vi "sedSpectrometer_acceptCommand_setSpectTempSetpoint.vi"(8 "error in (no error)":errorcluster, 11 "command_setSpectTempSetpoint_Ctl":T1) -> (0 "error out":errorcluster, 2 "function return":i32, 3 "command_setSpectTempSetpoint_Ctl out":T1)   [LabVIEW 2016, in "SALLV_sedSpectrometer.lvlib"]
doc: "int sedSpectrometer_shm_acceptCommand_setSpectTempSetpointLV(sedSpectrometer_command_setSpectTempSetpointLV *command_setSpectTempSetpoint_Ctl );"
uses:
  SALLV_sedSpectrometer.lvlib
  DataTypes/command_setSpectTempSetpoint.ctl
  SALLV_sedSpectrometer.so
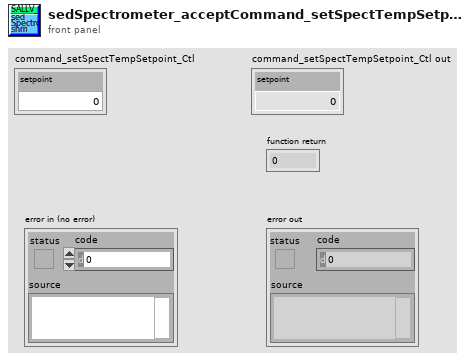
[diagram p1: front panel]
types:
  T1 = typedef "SALLV_sedSpectrometer.lvlib/command_setSpectTempSetpoint.ctl" = cluster{"setpoint":sgl}
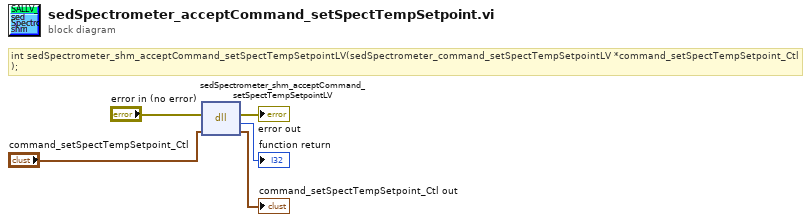
[diagram p0: block diagram]
diagram:
  # "int sedSpectrometer_shm_acceptCommand_setSpectTempSetpointLV(sedSpectrometer_command_setSpectTempSetpointLV *command_setSpectTempSetpoint_Ctl );"
  n1 = dll-call lib="home/harini/TCS/ts_sallv_sedSpectrometer/SALLV_sedSpectrometer.*" fn="sedSpectrometer_shm_acceptCommand_setSpectTempSetpointLV"(error in="error in (no error)", "command_setSpectTempSetpoint_Ctl"="command_setSpectTempSetpoint_Ctl") -> (error out=→"error out":errorcluster, →"function return":i32, "command_setSpectTempSetpoint_Ctl"=→"command_setSpectTempSetpoint_Ctl out":T1)  [unwired: 2 in, 1 out]
